vi "sv_Total Band Power for Octave (1 Ch).vi"(0 "octave spectrum":T5 {"band power [dB EU]" format="%.2f"; "nominal frequencies [Hz]" format="%.2f"}, 9 "octave info":T1={"standard"=enum."ANSI S1.11", "bandwidth"=enum."1 octave", "low band"=0, "high band"=0, "weighting filter"=0, "dB reference"=0.0, "dB On"=FALSE, "unit label"="", "channel name"="", "description"="", "engineering units"=1, "custom label"="", "spectrum type"=enum."magnitude", "spectral density"=FALSE, "filters settled"=FALSE} {"engineering units" items=["custom..."=0, "V"=1, "A"=21, "C"=30, "pC"=31, "s"=32, "-"=29, "Pa"=2, "N"=20, "g"=3, "m/s^2"=4, "m/s"=5, "m"=6, "mm/s"=12, "mm"=13, "micron/s"=14, "micron"=15, "in/s^2"=7, "in/s"=8, "in"=9, "mil/s"=10, "mil"=11, "rad/s^2"=16, "rad/s"=17, "rad"=18, "deg/s^2"=26, "deg/s"=27, "deg"=28, "RPM"=22, "cycle/s^2"=23, "Hz"=24, "cycle"=25, "strain"=19]; "dB reference" format="%.2e"; "weighting filter" items=["Linear", "A-weighting", "B-weighting", "C-weighting", "ITU-R 468-4", "Dolby", "CCITT", "C-message", "Wb", "Wc", "Wd", "We", "Wf", "Wh", "Wj", "Wk", "Wm", "AES17 20 kHz lowpass", "AES17 40 kHz lowpass", "AES17 20 kHz highpass", "AES17 40 kHz highpass"]}, 11 "error in (no error)":errorcluster) -> (4 "dup octave spectrum":T5 {"band power [dB EU]" format="%.2f"; "nominal frequencies [Hz]" format="%.2f"}, 6 "unit label":string, 10 "dup octave info":T1={"standard"=enum."ANSI S1.11", "bandwidth"=enum."1 octave", "low band"=0, "high band"=0, "weighting filter"=0, "dB reference"=0.0, "dB On"=FALSE, "unit label"="", "channel name"="", "description"="", "engineering units"=1, "custom label"="", "spectrum type"=enum."magnitude", "spectral density"=FALSE, "filters settled"=FALSE} {"engineering units" items=["custom..."=0, "V"=1, "A"=21, "C"=30, "pC"=31, "s"=32, "-"=29, "Pa"=2, "N"=20, "g"=3, "m/s^2"=4, "m/s"=5, "m"=6, "mm/s"=12, "mm"=13, "micron/s"=14, "micron"=15, "in/s^2"=7, "in/s"=8, "in"=9, "mil/s"=10, "mil"=11, "rad/s^2"=16, "rad/s"=17, "rad"=18, "deg/s^2"=26, "deg/s"=27, "deg"=28, "RPM"=22, "cycle/s^2"=23, "Hz"=24, "cycle"=25, "strain"=19]; "dB reference" format="%.2e"; "weighting filter" items=["Linear", "A-weighting", "B-weighting", "C-weighting", "ITU-R 468-4", "Dolby", "CCITT", "C-message", "Wb", "Wc", "Wd", "We", "Wf", "Wh", "Wj", "Wk", "Wm", "AES17 20 kHz lowpass", "AES17 40 kHz lowpass", "AES17 20 kHz highpass", "AES17 40 kHz highpass"]}, 14 "total band power [dB EU]":dbl format="%.2f", 15 "error out":errorcluster)   [LabVIEW 2017, in "SoundVib_Octave.lvlib"]
uses:
  <vilib>/addons/Sound and Vibration/svt_Octave/SoundVib_Octave.lvlib
  <vilib>/addons/_NISVFA/_Shared subVIs/Controls/svc_Octave Info.ctl
  <vilib>/addons/_NISVFA/_Shared subVIs/Controls/svc_Octave Standard.ctl
  <vilib>/addons/_NISVFA/_Shared subVIs/Controls/svc_Weighting Filter Text Ring.ctl
  <vilib>/addons/_NISVFA/_Shared subVIs/Controls/svc_Engineering Units Text Ring.ctl
  <vilib>/addons/Sound and Vibration/svt_Octave_2014 standard/SoundVib_Octave_2014 standard.lvlib
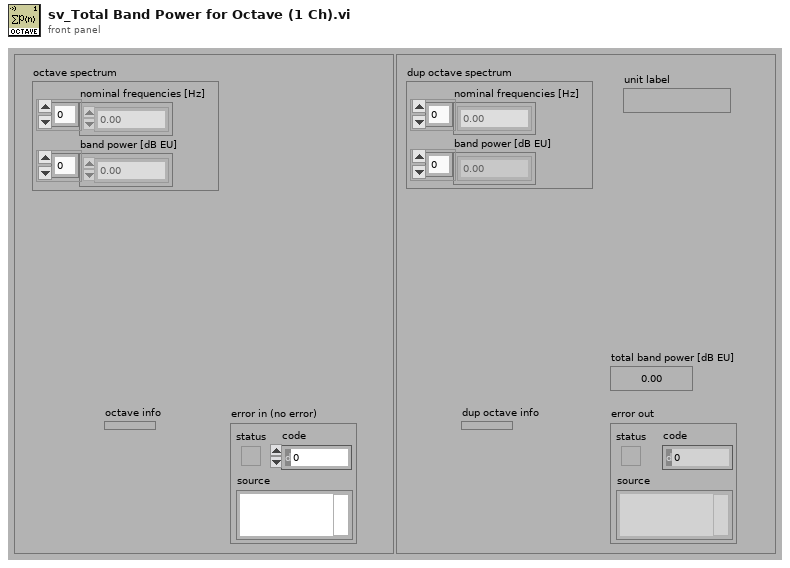
[diagram p1: front panel]
types:
  T1 = typedef "svc_Octave Info.ctl" = cluster{"standard":T2, "bandwidth":enum16{"1 octave", "1/3 octave", "1/6 octave", "1/12 octave", "1/24 octave"}, "low band":i32, "high band":i32, "weighting filter":T3, "dB reference":dbl, "dB On":bool, "unit label":string, "channel name":string, "description":string, "engineering units":T4, "custom label":string, "spectrum type":enum16{"power", "magnitude"}, "spectral density":bool, "filters settled":bool}
  T2 = typedef "svc_Octave Standard.ctl" = enum16{"ANSI S1.11", "IEC 61260"}
  T3 = typedef "svc_Weighting Filter Text Ring.ctl" = u16
  T4 = typedef "svc_Engineering Units Text Ring.ctl" = u16
  T5 = cluster{"nominal frequencies [Hz]":dbl[], "band power [dB EU]":dbl[]}
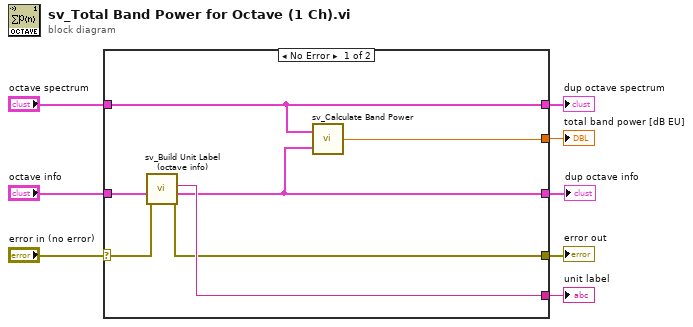
[diagram p0: block diagram]
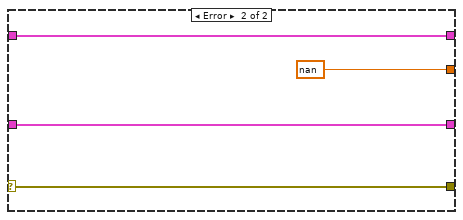
[diagram p2: hidden frame]
diagram:
  n1 = case shown="No Error" "error in (no error)" {
    selector: "error in (no error)" -> [w13 w18]
    tunnel: [w12 w18] -> w8
    tunnel: [w11 nan] -> w7
    tunnel: [w14 _] -> w6
    tunnel: "octave spectrum" -> [w10 w17]
    tunnel: [w10 w17] -> w3
    tunnel: "octave info" -> [w15 w16]
    tunnel: [w9 w16] -> w2
    frame No Error {
      n2 = call <vilib>:"sv_Build Unit Label (octave info).vi"("error in (no error)"=w13, "octave info"=w15) -> ("error out"=w12:errorcluster, "octave info out"=w9:T1, "unit label"=w14:string)  [unwired: 7 in]
      n3 = call <vilib>:"sv_Calculate Band Power.vi"("octave info"=w9, "octave spectrum"=w10) -> ("total band power"=w11:dbl)
    }
    frame Error {
    }
  }
  "error out" <- w8
  "total band power [dB EU]" <- w7
  "unit label" <- w6
  "dup octave spectrum" <- w3
  "dup octave info" <- w2
